vi "REPORT_CBATCH_save_pdf.vi"(8 "error_in":errorcluster) -> (0 "error_out":errorcluster)   [LabVIEW 2019]
uses:
  FGV/REPORTS_records_display/FGV_REPORTS_records_display.ctl
  typedef/REPORT_CBATCH_all_info.ctl
  DATES/typedef/REPORT_DATES_statuses.ctl
  <vilib>/Exaprom PDF/Controls/Image Controls/Image alignment and position.ctl
  <vilib>/Exaprom PDF/Controls/Image Controls/Image aligment.ctl
  <vilib>/Exaprom PDF/Controls/Table Controls/Row Predefined borders cluster.ctl
  <vilib>/Exaprom PDF/Controls/Table Controls/Row Predefined borders.ctl
  <vilib>/Exaprom PDF/Controls/Page Controls/Page setup.ctl
  <vilib>/Exaprom PDF/Controls/Page Controls/Page size.ctl
  <vilib>/Exaprom PDF/Controls/Page Controls/Page Orientation.ctl
  <vilib>/Exaprom PDF/Controls/Page Controls/Page Layout Custom.ctl
  <vilib>/Exaprom PDF/Controls/Page Controls/Page margins.ctl
  <vilib>/Exaprom PDF/Controls/Table Controls/Cell Font, type, Alignment and LS V2.ctl
  <vilib>/Exaprom PDF/Controls/Table Controls/Cell Type, Alignment and LS.ctl
  <vilib>/Exaprom PDF/Controls/Table Controls/Cell Alignment 20px.ctl
  <vilib>/Exaprom PDF/Controls/Table Controls/Text vertical arrangement.ctl
  <vilib>/Exaprom PDF/Controls/Text Controls/Line spacing.ctl
  <vilib>/Exaprom PDF/Controls/Font Controls/Font complete cluster.ctl
  <vilib>/Exaprom PDF/Controls/Font Controls/Font size.ctl
  <vilib>/Exaprom PDF/Controls/Font Controls/Font color.ctl
  <vilib>/Exaprom PDF/Controls/Font Controls/Type and encoding.ctl
  <vilib>/Exaprom PDF/Controls/Text Controls/Unicode/Type and run direction.ctl
  REPORT_font_for_pdf_report.ctl
  _misc/AULocalize/SubVIs/Get Localized Phrase Compact Interface 0D.vi
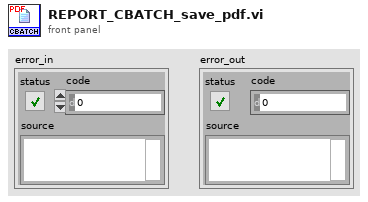
[diagram p1: front panel]
types:
  T1 = typedef "REPORT_CBATCH_all_info.ctl" = cluster{"batch_code":string, "records":string[][], "record_statuses":T2[], "column_headers":string[], "displayed_rows":string[][], "displayed_statuses":T2[], "column_widths":i16[], "active_page":i32}
  T2 = typedef "REPORT_DATES_statuses.ctl" = enum16{"GEAR_OK", "GEAR_NOK", "GEAR_interrupted", "GEAR_in_operation", "GEAR_unexpected"}
  T3 = typedef "FGV_REPORTS_records_display.ctl" = enum16{"initialize", "GEAR_set_serial", "GEAR_set_header", "GEAR_set_operations", "GEAR_set_results", "GEAR_set_batches", "GEAR_get_serial", "GEAR_get_operation_IDs", "GEAR_toggle_results", "GEAR_show_all_results", "GEAR_hide_all_results", "GEAR_display", "GEAR_filter", "GEAR_restore", "GEAR_clear", "GEAR_get_all_info", "DATES_set_dates", "DATES_set_gears", "DATES_display", "DATES_filter", "DATES_first_page", "DATES_previous_page", "DATES_next_page", "DATES_last_page", "DATES_restore", "DATES_clear", "DATES_get_all_info", "PBATCH_set_batch_no", "PBATCH_set_gears", "PBATCH_display", "PBATCH_filter", "PBATCH_first_page", "PBATCH_previous_page", "PBATCH_next_page", "PBATCH_last_page", "PBATCH_restore", "PBATCH_clear", "PBATCH_get_all_info", "OPRTN_set_OP", "OPRTN_set_dates", "OPRTN_set_gears", "OPRTN_set_hidden_columns", "OPRTN_display", "OPRTN_filter", "OPRTN_filter_no_page_reset", "OPRTN_first_page", "OPRTN_previous_page", "OPRTN_next_page", "OPRTN_last_page", "OPRTN_restore", "OPRTN_clear", "OPRTN_get_all_info", "CFG_set_type", "CFG_set_dates", "CFG_set_records", "CFG_display", "CFG_filter", "CFG_first_page", "CFG_previous_page", "CFG_next_page", "CFG_last_page", "CFG_restore", "CFG_clear", "CFG_get_all_info", "AUDIT_set_dates", "AUDIT_set_records", "AUDIT_display", "AUDIT_filter", "AUDIT_first_page", "AUDIT_previous_page", "AUDIT_next_page", "AUDIT_last_page", "AUDIT_restore", "AUDIT_clear", "AUDIT_get_all_info", "OKNOK_set_dates", "OKNOK_set_records", "OKNOK_display", "OKNOK_restore", "OKNOK_clear", "OKNOK_get_all_info", "REWORKS_set_dates", "REWORKS_set_from_to", "REWORKS_set_records", "REWORKS_display", "REWORKS_filter", "REWORKS_first_page", "REWORKS_previous_page", "REWORKS_next_page", "REWORKS_last_page", "REWORKS_restore", "REWORKS_clear", "REWORKS_get_all_info", "PACE_set_dates", "PACE_set_limits", "PACE_set_records", "PACE_display", "PACE_restore", "PACE_clear", "PACE_get_all_info", "CBATCH_set_code", "CBATCH_set_records", "CBATCH_display", "CBATCH_filter", "CBATCH_first_page", "CBATCH_previous_page", "CBATCH_next_page", "CBATCH_last_page", "CBATCH_restore", "CBATCH_clear", "CBATCH_get_all_info", "CMPNT_set_serial", "CMPNT_set_records", "CMPNT_display", "CMPNT_first_page", "CMPNT_previous_page", "CMPNT_next_page", "CMPNT_last_page", "CMPNT_restore", "CMPNT_clear", "CMPNT_get_all_info", "clear"}
  T4 = typedef "Cell Font, type, Alignment and LS V2.ctl" = cluster{"Cell Type, Alignment and LS":T5, "Font":T9}
  T5 = typedef "Cell Type, Alignment and LS.ctl" = cluster{"Cell Alignment":T6, "Text rotation":T7, "Line spacing":T8}
  T6 = typedef "Cell Alignment 20px.ctl" = u16
  T7 = typedef "Text vertical arrangement.ctl" = enum16{"None", "Clockwise", "Counterclockwise"}
  T8 = typedef "Line spacing.ctl" = enum16{"Select", "1.0", "1.5", "2.0"}
  T9 = typedef "Font complete cluster.ctl" = cluster{"Name":string, "Size":T10, "Color":T11, "Style":cluster{"Bold":bool, "Italic":bool, "Underline":bool, "Strikeout":bool}, "Type":T12}
  T10 = typedef "Font size.ctl" = sgl
  T11 = typedef "Font color.ctl" = u32
  T12 = typedef "Type and encoding.ctl" = cluster{"Type&direction":T13, "Embedded":bool, "Encoding":string}
  T13 = typedef "Type and run direction.ctl" = enum16{"Select", "ASCII", "UTF-16", "UTF-16 (default)", "UTF-16 (LTR)", "UTF-16 (RTL)"}
  T14 = typedef "Page setup.ctl" = cluster{"Page Size":T15, "Orientation":T16, "Custom Size":T17, "Margins":T18}
  T15 = typedef "Page size.ctl" = i32
  T16 = typedef "Page Orientation.ctl" = enum16{"Portrait", "Landscape"}
  T17 = typedef "Page Layout Custom.ctl" = cluster{"Width":sgl, "Height":sgl}
  T18 = typedef "Page margins.ctl" = cluster{"Left":sgl, "Right":sgl, "Top":sgl, "Bottom":sgl}
  T19 = cluster{"Font Name:":string, "Size":i16, "Strikeout?":bool, "Italic?":bool, "Underline?":bool, "Outline?":bool, "Shadow?":bool, "Bold?":bool}
  T20 = typedef "Row Predefined borders cluster.ctl" = cluster{"Borders":T21, "Header":cluster{"Thickness":sgl, "Line":u32, "Background ":u32}, "Data":cluster{"Thickness":sgl, "Line":u32, "Background ":u32}}
  T21 = typedef "Row Predefined borders.ctl" = u16
  T22 = typedef "Image alignment and position.ctl" = cluster{"Alignment":T23, "X ":sgl, "Y":sgl, "Indentation":sgl}
  T23 = typedef "Image aligment.ctl" = enum16{"Absolute (X,Y)", "Left", "Center", "Right", "Left (textwrap)", "Right (textwrap)"}
  T24 = typedef "REPORT_font_for_pdf_report.ctl" = cluster{"Name":string, "Size":T10, "Color":T11, "Style":cluster{"Bold":bool, "Italic":bool, "Underline":bool, "Strikeout":bool}, "Type":T12}
  T25 = typedef "Table Appearance and Font Row [ ].ctl" = T26[]
  T26 = typedef "One Row Appearance.ctl" = cluster{"Row":T27, "Cell [ ]":T28[]}
  T27 = typedef "Row from to.ctl" = cluster{"From #":i16, "to #":i16}
  T28 = typedef "Cell, Alignment, LS and Font - hide Vmerge.ctl" = cluster{"Text":T5, "Cell Appearance":T29, "HMerge":T31, "VMerge":T32, "Font":T9}
  T29 = typedef "Cell Appearance.ctl" = cluster{"Border":T30, "Thickness":sgl, "Color":u32, "BG":u32}
  T30 = typedef "Cell Border 20 px.ctl" = u16
  T31 = typedef "Merge Horizontal.ctl" = cluster{"From":i8, "to":i8}
  T32 = typedef "Merge Vertical.ctl" = cluster{"From":i8, "to":i8}
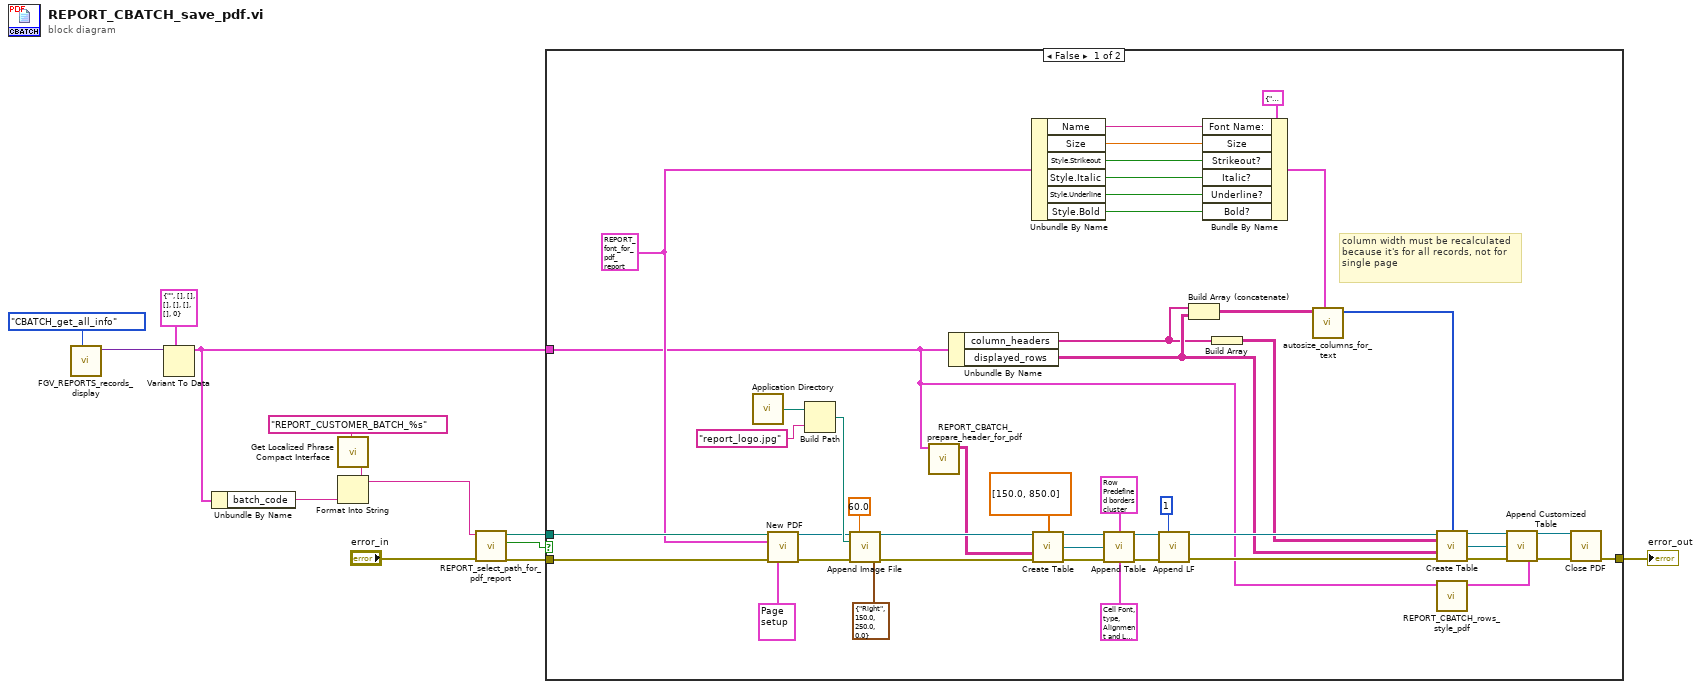
[diagram p0: block diagram]
diagram:
  n1 = call "FGV_REPORTS_records_display.vi"("options"=FGV_REPORTS_records_display."CBATCH_get_all_info") -> ("output"=w13:variant)  [unwired: 9 in, 1 out]
  n2 = Variant To Data(type=T1 {"batch_code"="", "records"=[], "record_statuses"=[], "column_headers"=[], "displayed_rows"=[], "displayed_statuses"=[], "column_widths"=[], "active_page"=0} ("REPORT_CBATCH_all_info"), Variant=w13) -> (data=w4:T1)  [unwired: 1 in, 1 out]
  n3 = Unbundle By Name(w4) -> ("batch_code"=w6:string)
  n4 = call-poly "Get Localized Phrase Compact Interface.vi"("Key"="REPORT_CUSTOMER_BATCH_%s" ("report_title")) -> ("Translated Phrase"=w1:string)
  n5 = Format Into String(format string=w1, w6) -> (resulting string=w5:string)  [unwired: 2 in, 1 out]
  n6 = call "REPORT_select_path_for_pdf_report.vi"("error_in"="error_in", "report_title"=w5) -> ("error_out"=w8:errorcluster, "cancelled"=w2:bool, "path_to_report"=w9:path)  [unwired: 7 in]
  n7 = case shown="False" w2 {
    tunnel: [w59 w60] -> w10
    tunnel: w9 -> [w58 _]
    tunnel: w8 -> [w57 w60]
    tunnel: w4 -> [w14 _]
    frame False {
      w23 = T24 {"Name"="Consolas", "Size"=10.0, "Color"=0, "Style"={"Bold"=FALSE, "Italic"=FALSE, "Underline"=FALSE, "Strikeout"=FALSE}, "Type"={"Type&direction"=enum."ASCII", "Embedded"=FALSE, "Encoding"="CP855"}} ("Default Font")
      # "column width must be recalculated because it's for all records, not for single page"
      n8 = call <vilib>:"Application Directory.vi"() -> ("Application Directory"=w51:path)
      n9 = call <vilib>:"New PDF.vi"("PDF Path"=w58, "Default Font"=w23, "error in (no error)"=w57, "Page Setup"=T14 {"Page Size"=11, "Orientation"=enum."Landscape", "Custom Size"={"Width"=216.0, "Height"=279.0}, "Margins"={"Left"=10.0, "Right"=10.0, "Top"=10.0, "Bottom"=10.0}}) -> ("PDF Report"=w45:refnum<class "PDF Report Class.lvclass">, "error out"=w46:errorcluster)  [unwired: 7 in, 3 out]
      n10 = Build Path(base path=w51, name or relative path="report_logo.jpg") -> (appended path=w47:path)
      n11 = call <vilib>:"Append Image File.vi"("PDF Report IN"=w45, "Scale (%)"=sgl 60.0, "Image path"=w47, "error in (no error)"=w46, "Position and indentation"=T22 {"Alignment"=enum."Right", "X "=150.0, "Y"=250.0, "Indentation"=0.0}) -> ("PDF Report OUT"=w30:refnum<class "PDF Report Class.lvclass">, "error out"=w29:errorcluster)  [unwired: 7 in, 2 out]
      n12 = call "REPORT_CBATCH_prepare_header_for_pdf.vi"("REPORT_CBATCH_all_info"=w14) -> ("report_header"=w28:string[][])  [unwired: 10 in]
      n13 = Unbundle By Name(w14) -> ("column_headers"=w26:string[], "displayed_rows"=w27:string[][])
      n14 = Unbundle By Name(w23) -> ("Name"=w20:string, "Size"=w19:T10, "Style.Strikeout"=w18:bool, "Style.Italic"=w17:bool, "Style.Underline"=w16:bool, "Style.Bold"=w15:bool)
      n15 = call <vilib>:"Create Table.vi"("PDF Report IN"=w30, "Table columnWidth [ ]"=sgl[] [150.0, 850.0], "Text Data 2D [ ]"=w28, "error in (no error)"=w29) -> ("PDF Report duplicate"=w38:refnum<class "PDF Report Class.lvclass">, "PDF Table"=w37:refnum<class "Pdfp Table Class.lvclass">, "error out"=w36:errorcluster)  [unwired: 9 in]
      n16 = call <vilib>:"Append Table.vi"("PDF Report IN"=w38, "Predefined Borders"=T20 {"Borders"=0, "Header"={"Thickness"=0.0, "Line"=0, "Background "=16777215}, "Data"={"Thickness"=0.0, "Line"=0, "Background "=16777215}}, "PDF Table"=w37, "error in (no error)"=w36, "Datas format"=T4 {"Cell Type, Alignment and LS"={"Cell Alignment"=0, "Text rotation"=enum."None", "Line spacing"=enum."Select"}, "Font"={"Name"="Consolas", "Size"=-1.0, "Color"=0, "Style"={"Bold"=FALSE, "Italic"=FALSE, "Underline"=FALSE, "Strikeout"=FALSE}, "Type"={"Type&direction"=enum."Select", "Embedded"=FALSE, "Encoding"=""}}}) -> ("PDF Report OUT"=w35:refnum<class "PDF Report Class.lvclass">, "error out"=w34:errorcluster)  [unwired: 9 in]
      n17 = call <vilib>:"Append LF.vi"("PDF Report IN"=w35, "Number of LF (default 1)"=u8 1, "error in (no error)"=w34) -> ("PDF Report duplicate"=w43:refnum<class "PDF Report Class.lvclass">, "error out"=w42:errorcluster)  [unwired: 11 in]
      n18 = Build Array (concatenate)(w26, w27) -> (w25:string[][])
      n19 = Bundle By Name(cluster=T19 {"Font Name:"="", "Size"=0, "Strikeout?"=FALSE, "Italic?"=FALSE, "Underline?"=FALSE, "Outline?"=FALSE, "Shadow?"=FALSE, "Bold?"=FALSE} ("font"), "Font Name:"=w20, "Size"=w19, "Strikeout?"=w18, "Italic?"=w17, "Underline?"=w16, "Bold?"=w15) -> (w22:T19)
      n20 = Build Array(w26) -> (w40:string[][])
      n21 = call "autosize_columns_for_text.vi"("font"=w22, "array_to_autosize"=w25) -> ("column_widths"=w24:i16[])  [unwired: 9 in]
      n22 = call <vilib>:"Create Table.vi"("PDF Report IN"=w43, "Table columnWidth [ ]"=w24, "Column Headers 2D [ ]"=w40, "Text Data 2D [ ]"=w27, "error in (no error)"=w42) -> ("PDF Report duplicate"=w41:refnum<class "PDF Report Class.lvclass">, "PDF Table"=w53:refnum<class "Pdfp Table Class.lvclass">, "error out"=w56:errorcluster)  [unwired: 8 in]
      n23 = call "REPORT_CBATCH_rows_style_pdf.vi"("REPORT_CBATCH_all_info"=w14) -> ("Row  [ ]"=w39:T25)  [unwired: 10 in]
      n24 = call <vilib>:"Append Customized Table.vi"("PDF Report IN"=w41, "PDF Table"=w53, "error in (no error)"=w56, "Row  [ ]"=w39) -> ("PDF Report OUT"=w54:refnum<class "PDF Report Class.lvclass">, "error out"=w55:errorcluster)  [unwired: 10 in]
      n25 = call <vilib>:"Close PDF.vi"("PDF Report"=w54, "error in (no error)"=w55) -> ("error out"=w59:errorcluster)  [unwired: 12 in, 1 out]
    }
    frame True {
    }
  }
  "error_out" <- w10
